vi "SECoP-deleteNode.vi"(8 "error in (no error)":errorcluster, 10 "node id":string, 11 "DLL path (in)":T1) -> (0 "error out":errorcluster, 3 "DLL path (out)":T1)   [LabVIEW 2023, in "SECoP.lvlib"]
doc: "Call <b>\"SECoP-deleteNode.vi\"</b> to delete an existing SECoP node. Any connected clients will be disconnected.\n\n<b>DLL path</b> input and output of cluster from \"SECoP-Initialize.vi\"\n<b>node id</b> unique name of the SECoP node"
uses:
  SECoP.lvlib
  SECoP-libraries.ctl
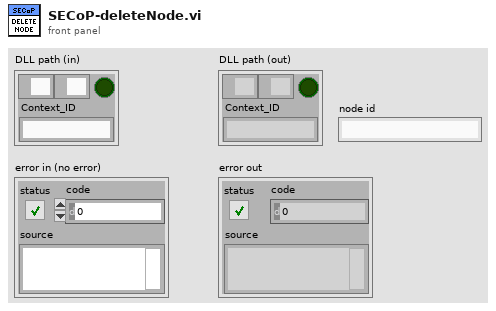
[diagram p1: front panel]
types:
  T1 = typedef "SECoP.lvlib/SECoP-libraries.ctl" = cluster{"serverDLL":path, "variantDLL":path, "cleanup_mode":bool, "Context_ID":string}
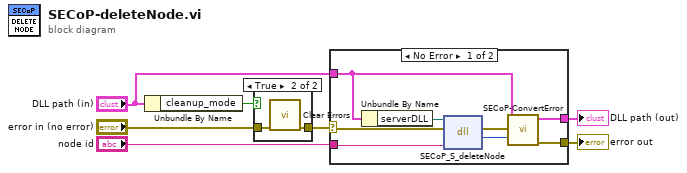
[diagram p0: block diagram]
diagram:
  n1 = Unbundle By Name("DLL path (in)") -> ("cleanup_mode"=w4:bool)
  n2 = case shown="True" w4 {
    tunnel: "error in (no error)" -> [w8 w10]
    tunnel: [w8 w9] -> w2
    frame False {
    }
    frame True {
      n3 = call <vilib>:"Clear Errors.vi"("error in (no error)"=w10) -> ("error out"=w9:errorcluster)  [unwired: 5 in, 1 out]
    }
  }
  n4 = case shown="No Error" w2 {
    selector: w2 -> [w14 w19]
    tunnel: "DLL path (in)" -> [w12 w20]
    tunnel: [w17 w20] -> w7
    tunnel: [w18 w19] -> w6
    tunnel: "node id" -> [w15 _]
    frame No Error {
      n5 = Unbundle By Name(w12) -> ("serverDLL"=w11:path)
      n6 = dll-call lib="Z:/Praktische Aufgaben/SECoP-LabVIEW2015/32bit/SECoP32.dll" fn="SECoP_S_deleteNode"(path in=w11, error in=w14, "node ID"=w15) -> (error out=w13:errorcluster, "return type"=w16:i32)  [unwired: 2 in, 1 out]
      n7 = call "SECoP-ConvertError.vi"("return code"=w16, "error in (no error)"=w13, "DLL path (in)"=w12) -> ("error out"=w18:errorcluster, "DLL path (out)"=w17:T1)  [unwired: 7 in]
    }
    frame Error {
    }
  }
  "DLL path (out)" <- w7
  "error out" <- w6
